vi "AlliGator Update Settings IRF Analysis Method Control.vi"(8 "error in (no error)":errorcluster, 11 "IRF Analysis Method Refnum":refnum<vi>) -> (0 "error out":errorcluster, 1 "Message":string)   [LabVIEW 2021, in "AlliGator Settings.lvlib"]
doc: "Update decay shifting parameters in the Settings window."
uses:
  AlliGator Settings.lvlib
  Graphs/XY Graph/XY Graph Plot Shift Method.ctl
  Graphs/XY Graph/XY Graph Add-Ons.lvlib
panel:
  # "see the AlliGator License on the block diagram (Ctrl+E or Window:Show Block Diagram)"
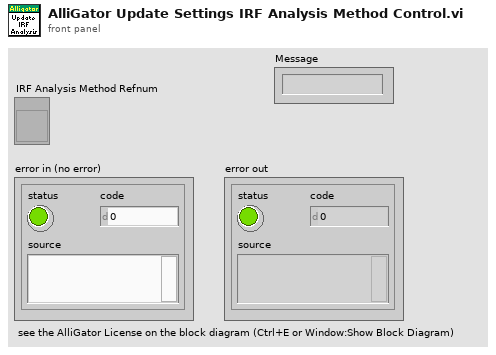
[diagram p1: front panel]
types:
  T1 = typedef "XY Graph Add-Ons.lvlib/XY Graph Plot Shift Method.ctl" = enum16{"Default", "CFD", "Threshold", "Cross-Correlation"}
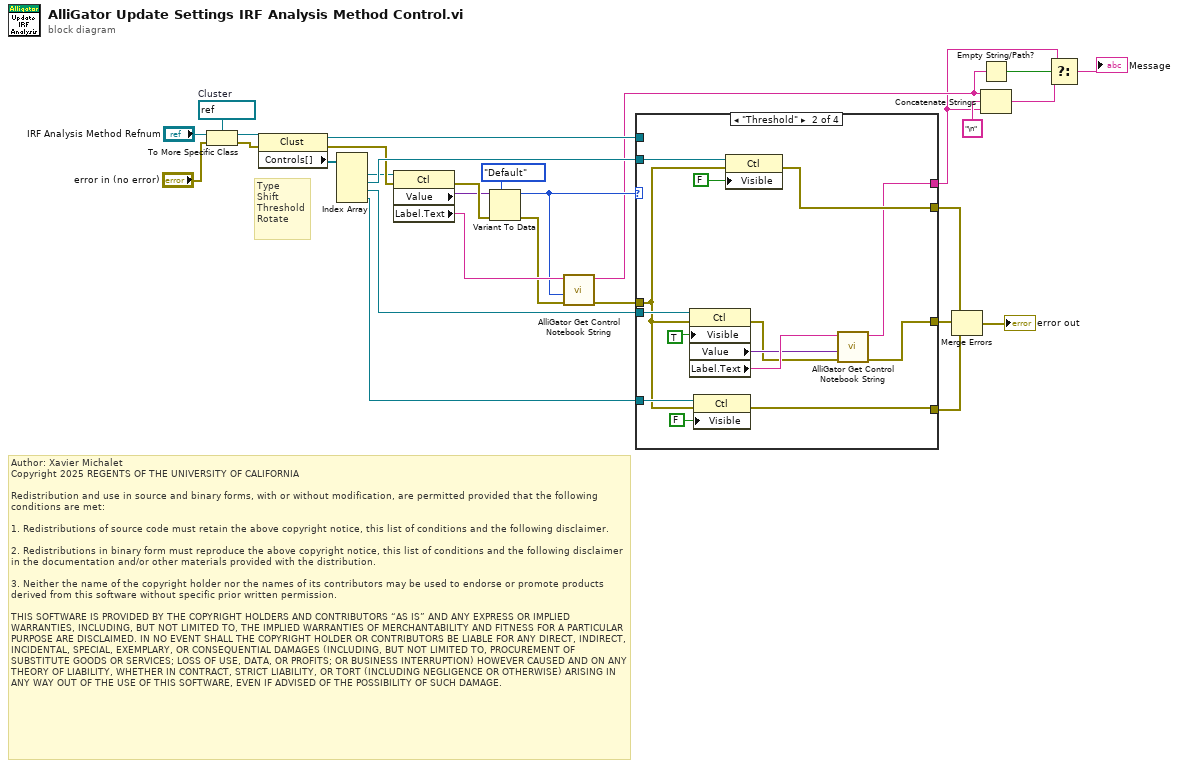
[diagram p0: block diagram]
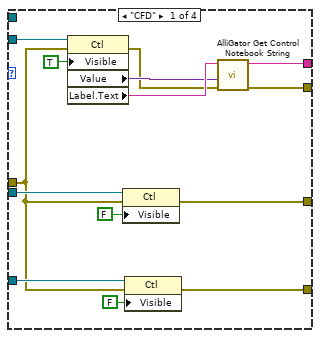
[diagram p2: hidden frame]
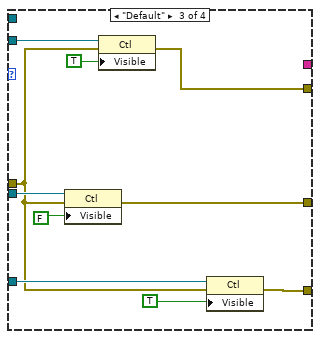
[diagram p3: hidden frame]
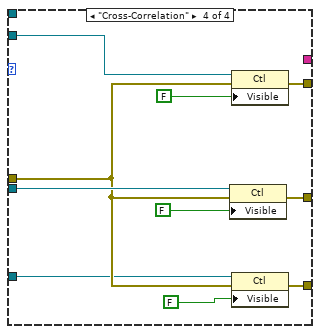
[diagram p4: hidden frame]
diagram:
  w19 = refnum<vi> refnum  # Cluster
  # "Author: Xavier Michalet\nCopyright 2025 REGENTS OF THE UNIVERSITY OF CALIFORNIA\n\nRedistribution and use in source and binary forms, with or without modification, are permitted provided that the following conditions are met:\n\n1. Redistributions of source code must retain the above copyright notice, this list of conditions and the following disclaimer.\n\n2. Redistributions in binary form must reproduce the above copyright notice, this list of conditions and the following disclaimer in the documentation and/or other materials provided with the distribution.\n\n3. Neither the name of the copyright holder nor the names of its contributors may be used to endorse or promote products derived from this software without specific prior written permission.\n\nTHIS SOFTWARE IS PROVIDED BY THE COPYRIGHT HOLDERS AND CONTRIBUTORS “AS IS” AND ANY EXPRESS OR IMPLIED WARRANTIES, INCLUDING, BUT NOT LIMITED TO, THE IMPLIED WARRANTIES OF MERCHANTABILITY AND FITNESS FOR A PARTICULAR PURPOSE ARE DISCLAIMED. IN NO EVENT SHALL THE COPYRIGHT HOLDER OR CONTRIBUTORS BE LIABLE FOR ANY DIRECT, INDIRECT, INCIDENTAL, SPECIAL, EXEMPLARY, OR CONSEQUENTIAL DAMAGES (INCLUDING, BUT NOT LIMITED TO, PROCUREMENT OF SUBSTITUTE GOODS OR SERVICES; LOSS OF USE, DATA, OR PROFITS; OR BUSINESS INTERRUPTION) HOWEVER CAUSED AND ON ANY THEORY OF LIABILITY, WHETHER IN CONTRACT, STRICT LIABILITY, OR TORT (INCLUDING NEGLIGENCE OR OTHERWISE) ARISING IN ANY WAY OUT OF THE USE OF THIS SOFTWARE, EVEN IF ADVISED OF THE POSSIBILITY OF SUCH DAMAGE."
  # "Type\nShift\nThreshold\nRotate"
  n1 = To More Specific Class(target class=w19, reference="IRF Analysis Method Refnum", error in="error in (no error)") -> (specific class reference=w18:refnum<vi>, error out=w10:errorcluster)
  n2 = property class="Clust"(reference=w18, error in=w10) -> (reference out=w16:refnum<vi>, error out=w22:errorcluster, "Controls[]"=w20:refnum<vi>[])
  n3 = Index Array(array=w20) -> (element #1=w21:refnum<vi>, element #2=w24:refnum<vi>, element #3=w25:refnum<vi>, element #4=w9:refnum<vi>)  [unwired: 4 in]
  n4 = property class="Ctl"(reference=w21, error in=w22) -> (error out=w26:errorcluster, "Value"=w23:variant, "Label.Text"=w15:string)  [unwired: 1 out]
  n5 = Variant To Data(error in=w26, type=XY_Graph_Plot_Shift_Method."Default" ("IRF Analysis Method"), Variant=w23) -> (data=w14:T1, error out=w13:errorcluster)
  n6 = call "AlliGator Get Control Notebook String.vi"("error in (no error)"=w13, "Value"=w14, "Control Label"=w15) -> ("error out"=w7:errorcluster, "Notebook String"=w5:string)  [unwired: 7 in]
  n7 = case shown="\"Threshold\"" w14 {
    tunnel: w24 -> [w43 w57 w67 w77]
    tunnel: w25 -> [w42 w56 w66 w76]
    tunnel: [w31 w53 w63 w73] -> w27
    tunnel: [w39 w44 w62 w72] -> w28
    tunnel: w16 -> [_ _ _ _]
    tunnel: w7 -> [w34 w46 w59 w71]
    tunnel: w9 -> [w35 w49 w61 w68]
    tunnel: [w33 w47 w58 w69] -> w8
    tunnel: [w30 w45 _ _] -> w3
    frame "CFD" {
      n8 = property class="Ctl"(reference=w43, error in=w34, "Visible"=TRUE) -> (error out=w32:errorcluster, "Value"=w37:variant, "Label.Text"=w38:string)  [unwired: 1 out]
      n9 = property class="Ctl"(reference=w42, error in=w34, "Visible"=FALSE) -> (error out=w39:errorcluster)  [unwired: 1 out]
      n10 = property class="Ctl"(reference=w35, error in=w34, "Visible"=FALSE) -> (error out=w33:errorcluster)  [unwired: 1 out]
      n11 = call "AlliGator Get Control Notebook String.vi"("error in (no error)"=w32, "Value"=w37, "Control Label"=w38) -> ("error out"=w31:errorcluster, "Notebook String"=w30:string)  [unwired: 7 in]
    }
    frame "Threshold" {
      n12 = property class="Ctl"(reference=w56, error in=w46, "Visible"=TRUE) -> (error out=w50:errorcluster, "Value"=w51:variant, "Label.Text"=w52:string)  [unwired: 1 out]
      n13 = property class="Ctl"(reference=w49, error in=w46, "Visible"=FALSE) -> (error out=w47:errorcluster)  [unwired: 1 out]
      n14 = property class="Ctl"(reference=w57, error in=w46, "Visible"=FALSE) -> (error out=w53:errorcluster)  [unwired: 1 out]
      n15 = call "AlliGator Get Control Notebook String.vi"("error in (no error)"=w50, "Value"=w51, "Control Label"=w52) -> ("error out"=w44:errorcluster, "Notebook String"=w45:string)  [unwired: 7 in]
    }
    frame "Default" {
      n16 = property class="Ctl"(reference=w66, error in=w59, "Visible"=FALSE) -> (error out=w62:errorcluster)  [unwired: 1 out]
      n17 = property class="Ctl"(reference=w67, error in=w59, "Visible"=TRUE) -> (error out=w63:errorcluster)  [unwired: 1 out]
      n18 = property class="Ctl"(reference=w61, error in=w59, "Visible"=TRUE) -> (error out=w58:errorcluster)  [unwired: 1 out]
    }
    frame "Cross-Correlation" {
      n19 = property class="Ctl"(reference=w76, error in=w71, "Visible"=FALSE) -> (error out=w72:errorcluster)  [unwired: 1 out]
      n20 = property class="Ctl"(reference=w77, error in=w71, "Visible"=FALSE) -> (error out=w73:errorcluster)  [unwired: 1 out]
      n21 = property class="Ctl"(reference=w68, error in=w71, "Visible"=FALSE) -> (error out=w69:errorcluster)  [unwired: 1 out]
    }
  }
  n22 = Merge Errors(w27, w28, w8) -> (→"error out":errorcluster)
  n23 = Empty String/Path?(string/path=w5) -> (empty?=w4:bool)
  n24 = Concatenate Strings(w5, "\n" ("string"), w3) -> (w2:string)
  n25 = Select(t=w3, s=w4, f=w2) -> (s? t:f=→"Message":string)
